vi "sub_slope2deg.vi"(11 "slope":dbl) -> (3 "deg":dbl)   [LabVIEW 2018]
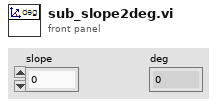
[diagram p1: front panel]
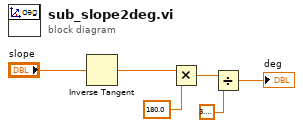
[diagram p0: block diagram]
diagram:
  n1 = Inverse Tangent(1:"slope") -> (0:w5:dbl)
  n2 = Multiply(x=w5, y=180.0) -> (x*y=w2:dbl)
  n3 = Divide(x=w2, y=3.141592653589793) -> (x/y=→"deg":dbl)
